vi "Connect.vi"(8 "error in":errorcluster) -> (0 "error out":errorcluster, 3 "UdsHandleOut":T1)   [LabVIEW 2011, in "Konvolucio MUDS150628.lvlib"]
uses:
  <instrlib>/Konvolucio MUDS150628/Konvolucio MUDS150628.lvlib
  <instrlib>/Konvolucio MUDS150628/Types/UdsHandleType.ctl
  <instrlib>/Konvolucio MCAN120803/Types/MCanHandleType.ctl
  C:/Program Files/National Instruments/LabVIEW 2011/instr.lib/Konvolucio MCAN120803/Private/Konvolucio.MCAN120803.dll
  Konvolucio MCAN120803/Private/Konvolucio.MCAN120803.dll
  <instrlib>/Konvolucio MCAN120803/Konvolucio MCAN120803.lvlib
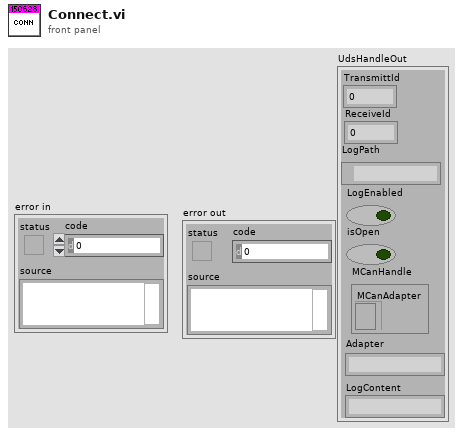
[diagram p1: front panel]
types:
  T1 = typedef "Konvolucio MUDS150628.lvlib/UdsHandleType.ctl" = cluster{"LogPath":path, "LogEnabled":bool, "isOpen":bool, "LogContent":string, "Adapter":string, "MCanHandle":T2, "TransmittId":u32, "ReceiveId":u32}
  T2 = typedef "Konvolucio MCAN120803.lvlib/MCanHandleType.ctl" = cluster{"MCanAdapter":refnum<k24>}
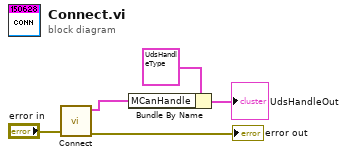
[diagram p0: block diagram]
diagram:
  n1 = call <instrlib>:"Connect.vi"("error in"="error in") -> ("error out"=→"error out":errorcluster, "MCanHandleOut"=w1:T2)  [unwired: 9 in]
  n2 = Bundle By Name(cluster=T1 {"LogPath"=path "", "LogEnabled"=FALSE, "isOpen"=FALSE, "LogContent"="", "Adapter"="", "MCanHandle"={"MCanAdapter"=refnum}, "TransmittId"=0, "ReceiveId"=0} ("UdsHandleOut"), "MCanHandle"=w1) -> (→"UdsHandleOut":T1)
